vi "LS_DAQ_Host.vi"() -> ()   [LabVIEW 2020]
panel:
  out "Temperature [°C]":dbl format="%#_3g"
  in  "Log data":bool
  out "Pulse count":dbl
  out "Frequency [Hz]":dbl
  in  "stop":bool
  out "Waveform Chart":cluster{"Numeric":dbl, "Numeric":dbl}(graph)
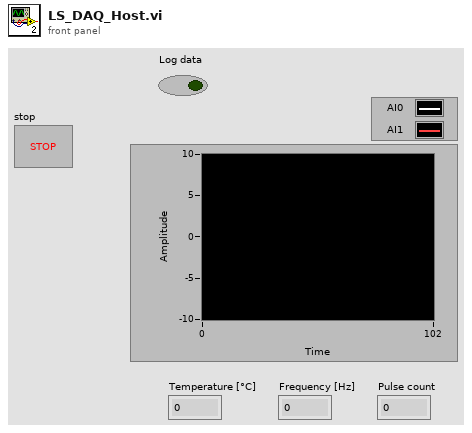
[diagram p1: front panel]
types:
  T1 = enum16{"open", "replace", "create", "open or create", "replace or create", "replace or create with confirmation"}
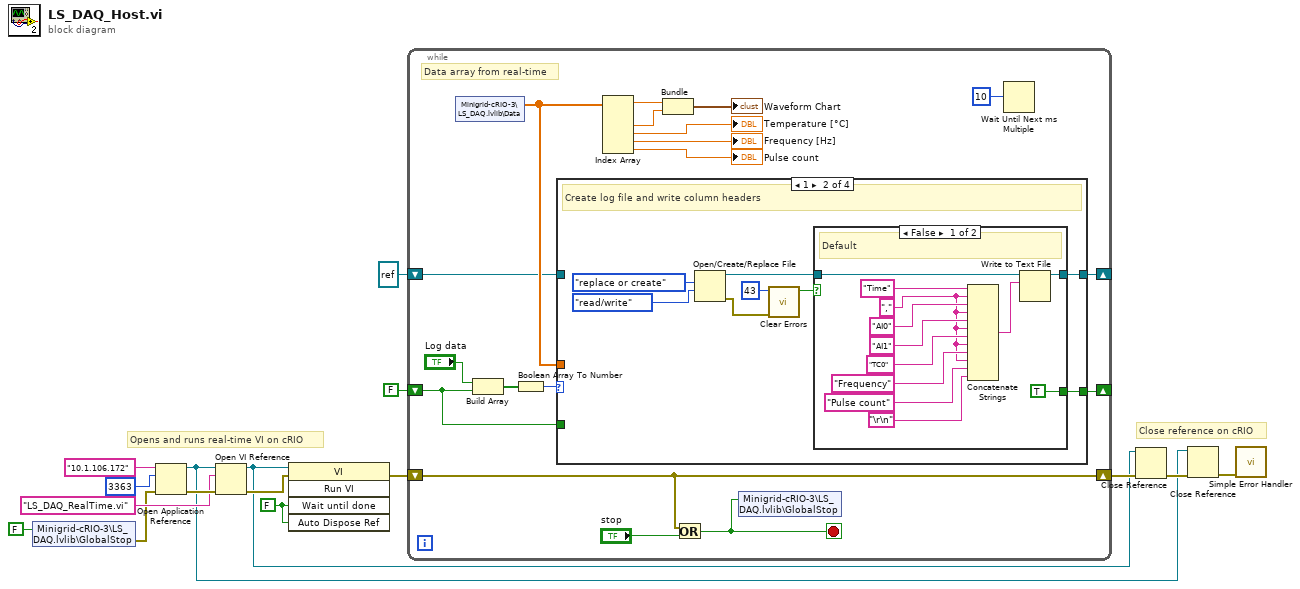
[diagram p0: block diagram]
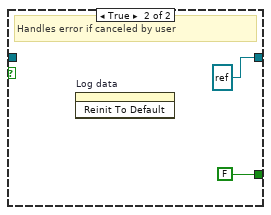
[diagram p3: hidden frame]
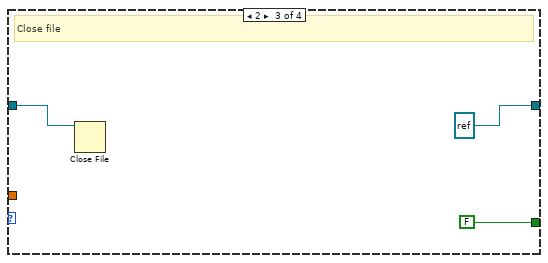
[diagram p4: hidden frame]
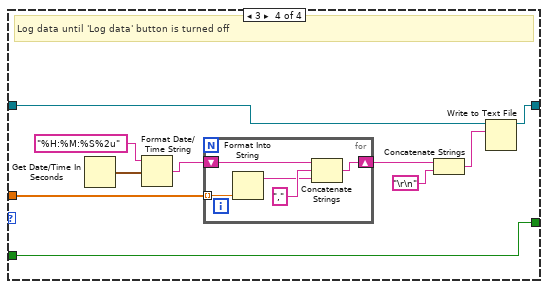
[diagram p5: hidden frame]
diagram:
  w1 = FALSE ("Wait Until Done")
  # "Close reference on cRIO"
  # "Opens and runs real-time VI on cRIO"
  n1 = shared-variable "Minigrid-cRIO-3\\LS_DAQ.lvlib\\GlobalStop"(FALSE ("GlobalStop")) -> (error out=w2:errorcluster)  [unwired: 1 in]
  n2 = Open Application Reference(8:w2, 10:u16 3363 ("port number or service name (3363)"), 11:"10.1.106.172" ("machine name (\"\":  open local reference)")) -> (0:w14:errorcluster, 3:w7:refnum<vi>)  [unwired: 1 in]
  n3 = Open VI Reference(application reference (local)=w7, vi path="LS_DAQ_RealTime.vi" ("machine name (\"\":  open local reference)"), error in (no error)=w14) -> (vi reference=w9:refnum<vi>, error out=w13:errorcluster)  [unwired: 3 in]
  n4 = invoke class="VI" method="Run VI"(reference=w9, error in=w13, "Wait until done"=w1, "Auto Dispose Ref"=w1) -> (error out=w12:errorcluster)  [unwired: 1 in, 4 out]
  n5 = while {
    shift-right: [w30] -> w10
    shift-left: w12 -> [w30]
    shift-right: [w23] -> _
    shift-left: FALSE -> [w22]
    shift-right: [w25] -> _
    shift-left: refnum<file> refnum ("refnum out") -> [w21]
    stop <- w29 stop-if-true
    # "Data array from real-time"
    n6 = shared-variable "Minigrid-cRIO-3\\LS_DAQ.lvlib\\Data"() -> (w24:dbl[])  [unwired: 1 in, 1 out]
    n7 = Build Array("Log data", w22) -> (w26:bool[])
    n8 = Boolean Array To Number(Boolean array=w26) -> (number=w28:u32)
    n9 = case shown="1" w28 {
      tunnel: [w35 w41 refnum<file> refnum ("refnum out") w66] -> w25
      tunnel: w24 -> [_ _ _ w70]
      tunnel: [w36 w40 FALSE w65] -> w23
      tunnel: w22 -> [w36 _ _ w65]
      tunnel: w21 -> [w35 _ w61 w71]
      frame 0, Default {
      }
      frame 1 {
        # "Create log file and write column headers"
        n10 = Open/Create/Replace File(operation (0:open)=T1."replace or create", access (0:read/write)=enum16{"read/write", "read-only", "write-only"}."read/write") -> (refnum out=w42:refnum<file>, error out=w39:errorcluster)  [unwired: 4 in, 1 out]
        n11 = call <vilib>:"Clear Errors.vi"("error in (no error)"=w39, "specific error code to clear (0: all)"=43) -> ("specific error cleared?"=w37:bool)  [unwired: 4 in, 1 out]
        n12 = case shown="False" w37 {
          tunnel: w42 -> [w56 _]
          tunnel: [w55 refnum<file> refnum ("refnum out")] -> w41
          tunnel: [TRUE FALSE] -> w40
          frame False {
            w47 = "," ("string")
            # "Default"
            n13 = Concatenate Strings("Time" ("string"), w47, "AI0" ("string"), w47, "AI1" ("string"), w47, "TC0" ("string"), w47, "Frequency" ("string"), w47, "Pulse count" ("string"), "\r\n") -> (w51:string)
            n14 = Write to Text File(file (use dialog)=w56, text=w51) -> (refnum out=w55:refnum<file>)  [unwired: 2 in, 2 out]
          }
          frame True {
            # "Handles error if canceled by user"
            n15 = invoke on="Log data" class="Bool (strict)" method="Reinit To Default"() -> ()  [unwired: 3 in, 3 out]
          }
        }
      }
      frame 2 {
        # "Close file"
        n16 = Close File(refnum=w61) -> ()  [unwired: 1 in, 2 out]
      }
      frame 3 {
        # "Log data until 'Log data' button is turned off"
        n17 = Get Date/Time In Seconds() -> (seconds since 1Jan1904=w64:timestamp)
        n18 = Format Date/Time String(time format string (%c)="%H:%M:%S%2u", seconds (now)=w64) -> (date/time string=w62:string)  [unwired: 1 in]
        n19 = for {
          tunnel: w70 -> [w75] mode=indexing
          shift-right: [w72] -> w69
          shift-left: w62 -> [w76]
          n20 = Format Into String(w75) -> (resulting string=w73:string)  [unwired: 3 in, 1 out]
          n21 = Concatenate Strings(w76, "," ("string"), w73) -> (w72:string)
        }
        n22 = Concatenate Strings(w69, "\r\n") -> (w67:string)
        n23 = Write to Text File(file (use dialog)=w71, text=w67) -> (refnum out=w66:refnum<file>)  [unwired: 2 in, 2 out]
      }
    }
    n24 = Index Array(array=w24) -> (element #1=w34:dbl, element #2=w33:dbl, element #3=→"Temperature [°C]":dbl, element #4=→"Frequency [Hz]":dbl, element #5=→"Pulse count":dbl)  [unwired: 5 in]
    n25 = Bundle("Numeric"=w34, "Numeric"=w33) -> (→"Waveform Chart":cluster{"Numeric":dbl, "Numeric":dbl})  [unwired: 1 in]
    n26 = Or(x=w30, y="stop") -> (x .or. y?=w29:bool)
    n27 = shared-variable "Minigrid-cRIO-3\\LS_DAQ.lvlib\\GlobalStop"(w29) -> ()  [unwired: 1 in, 1 out]
    n28 = Wait Until Next ms Multiple(millisecond multiple=u32 10 ("milliseconds to wait")) -> ()  [unwired: 1 out]
  }
  n29 = Close Reference(reference=w9, error in (no error)=w10) -> (error out=w8:errorcluster)
  n30 = Close Reference(reference=w7, error in (no error)=w8) -> (error out=w6:errorcluster)
  n31 = call <vilib>:"Simple Error Handler.vi"("error in (no error)"=w6) -> ()  [unwired: 4 in, 5 out]
